vi "Ev Apply.vi"(8 "error in (no error)":errorcluster, 11 "IDE simple in":refnum<class "Main Panel.lvclass">) -> (0 "error out":errorcluster, 3 "IDE simple out":refnum<class "Main Panel.lvclass">)   [LabVIEW 2018, in "Main Panel.lvlib" / "Main Panel.lvclass"]
uses:
  Main Panel.lvclass
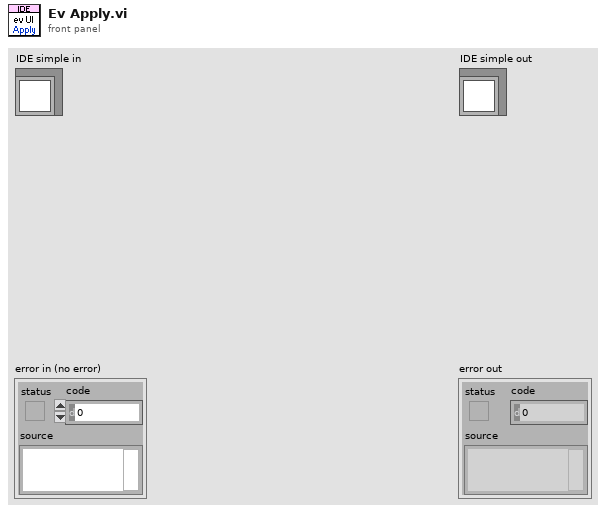
[diagram p1: front panel]
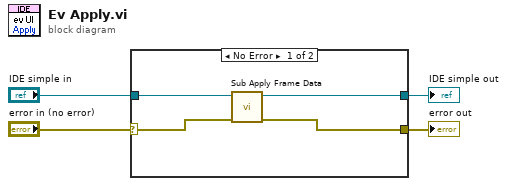
[diagram p0: block diagram]
diagram:
  n1 = case shown="No Error" "error in (no error)" {
    selector: "error in (no error)" -> [w7 w10]
    tunnel: [w5 w10] -> w3
    tunnel: [w6 w9] -> w1
    tunnel: "IDE simple in" -> [w8 w9]
    frame No Error {
      n2 = call "Sub Apply Frame Data.vi"("error in (no error)"=w7, "IDE simple in"=w8) -> ("error out"=w5:errorcluster, "IDE simple out"=w6:refnum<class "Main Panel.lvclass">)  [unwired: 8 in]
    }
    frame Error {
    }
  }
  "error out" <- w3
  "IDE simple out" <- w1
